vi "Timer_GetInternal.vi"(8 "Pass_Through_Time":dbl=-1.0 format="%33.4f", 11 "TIMER":T1 {"Accumulated TIme" format="%13.5p"; "StartTime" format="%13.5p"}) -> (1 "SystemTime":dbl, 3 "CurrentTImer":dbl)   [LabVIEW 2019, in "Trajectory_Library.lvlib"]
doc: "THIS IS AN INTERNAL ROUTINE. DO NOT USE.\n\n \nGet the current time from the timer. If the clock is running it is derived from the current system clock the start time stored in the timer class. If the clock is not running, then return the time when it was last stopped.\n\nInputs:\n - Timer -- The Timer data cluster\n\nOutputs:\n - CurrentTimer -- Current time value for this timer in seconds\n - SystemTimer -- Current system time"
uses:
  Trajectory_Library.lvlib
  TypeDef/TIMER.ctl
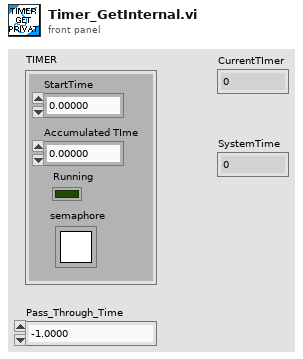
[diagram p1: front panel]
types:
  T1 = typedef "Trajectory_Library.lvlib/TIMER.ctl" = cluster{"StartTime":dbl, "Accumulated TIme":dbl, "Running":bool, "semaphore":T2}
  T2 = typedef "Semaphore RefNum" = refnum<k1>
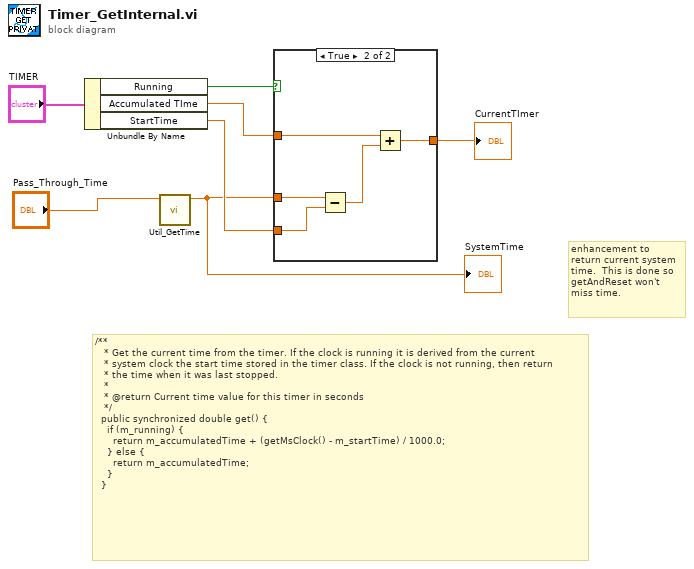
[diagram p0: block diagram]
diagram:
  # "enhancement to \nreturn current system\ntime.  This is done so \ngetAndReset won't\nmiss time."
  # "/**\n   * Get the current time from the timer. If the clock is running it is derived from the current\n   * system clock the start time stored in the timer class. If the clock is not running, then return\n   * the time when it was last stopped.\n   *\n   * @return Current time value for this timer in seconds\n   */\n  public synchronized double get() {\n    if (m_running) {\n      return m_accumulatedTime + (getMsClock() - m_startTime) / 1000.0;\n    } else {\n      return m_accumulatedTime;\n    }\n  }"
  n1 = Unbundle By Name("TIMER") -> ("Running"=w5:bool, "Accumulated TIme"=w4:dbl, "StartTime"=w3:dbl)
  n2 = call "Util_GetTime.vi"("Pass_Through_Time"="Pass_Through_Time") -> ("FPGA_Time_Seconds"=w2:dbl)  [unwired: 9 in, 1 out]
  "SystemTime" <- w2
  n3 = case shown="True" w5 {
    tunnel: w4 -> [w8 w11]
    tunnel: [w8 w12] -> w7
    tunnel: w3 -> [_ w13]
    tunnel: w2 -> [_ w9]
    frame False {
    }
    frame True {
      n4 = Subtract(x=w9, y=w13) -> (x-y=w10:dbl)
      n5 = Add(x=w11, y=w10) -> (x+y=w12:dbl)
    }
  }
  "CurrentTImer" <- w7
